vi "reset_trig.vi"(8 "error in (no error)":errorcluster, 11 "VISA resource name":refnum<visa-resource-name>) -> (0 "error out":errorcluster, 3 "VISA resource name out":refnum<visa-resource-name>)   [LabVIEW 2011]
doc: "This vi resets TRIG2 (DG645) to its defaultsetup and then configures a default setup for the chirped pulse setup.\nThis includes activating the burst mode (3 bursts, 100us burst period), setting polarities as well as setting all delays and durations to 0."
uses:
  global.vi
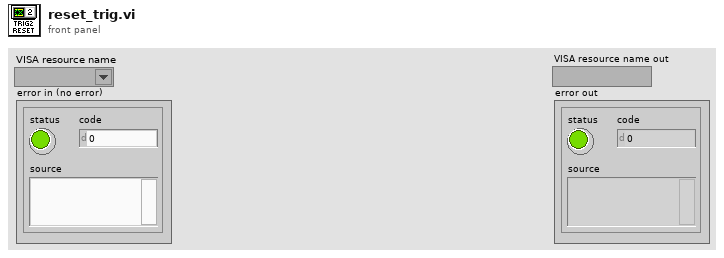
[diagram p1: front panel]
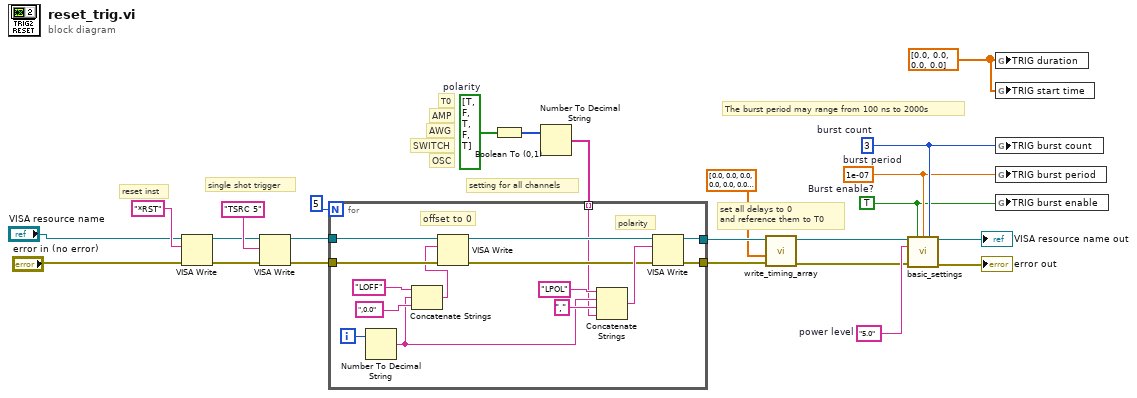
[diagram p0: block diagram]
diagram:
  w2 = bool[] [TRUE, FALSE, TRUE, FALSE, TRUE]  # polarity
  w5 = dbl[] [0.0, 0.0, 0.0, 0.0] ("duration")
  w12 = 3  # burst count
  w11 = 1e-07  # burst period
  w10 = TRUE  # Burst enable?
  w17 = "5.0"  # power level
  # "OSC"
  # "SWITCH"
  # "AWG"
  # "AMP"
  # "T0"
  # "The burst period may range from 100 ns to 2000s"
  # "set all delays to 0 \nand reference them to T0"
  # "reset inst"
  # "setting for all channels"
  # "single shot trigger"
  n1 = VISA Write(VISA resource name="VISA resource name", write buffer="*RST", error in (no error)="error in (no error)") -> (VISA resource name out=w19:refnum<visa-resource-name>, error out=w20:errorcluster)  [unwired: 1 out]
  n2 = VISA Write(VISA resource name=w19, write buffer="TSRC 5" ("Query 2"), error in (no error)=w20) -> (VISA resource name out=w22:refnum<visa-resource-name>, error out=w21:errorcluster)  [unwired: 1 out]
  n3 = Boolean To (0,1)(Boolean=w2) -> (0, 1=w3:i16[])
  n4 = Number To Decimal String(number=w3) -> (decimal integer string=w1:string[])  [unwired: 1 in]
  n5 = for {
    N: 5 -> [_]
    tunnel: w22 -> [w37]
    tunnel: [w28] -> w9
    tunnel: w21 -> [w36]
    tunnel: [w27] -> w8
    tunnel: w1 -> [w25] mode=indexing
    i -> [w35]
    # "polarity"
    # "offset to 0"
    n6 = Number To Decimal String(number=w35) -> (decimal integer string=w26:string)  [unwired: 1 in]
    n7 = Concatenate Strings("LOFF" ("Query 2"), w26, ",0.0" ("Query 2")) -> (w32:string)
    n8 = VISA Write(VISA resource name=w37, write buffer=w32, error in (no error)=w36) -> (VISA resource name out=w28:refnum<visa-resource-name>, error out=w27:errorcluster)  [unwired: 1 out]
    n9 = Concatenate Strings("LPOL" ("Query 2"), w26, "," ("string"), w25) -> (w30:string)
    n10 = VISA Write(VISA resource name=w28, write buffer=w30, error in (no error)=w27) -> ()  [unwired: 3 out]
  }
  n11 = call "write_timing_array.vi"("error in"=w8, "delay array"=dbl[] [0.0, 0.0, 0.0, 0.0, 0.0, 0.0, 0.0, 0.0] ("duration"), "VISA resource in"=w9) -> ("error out 2"=w6:errorcluster, "VISA resource out"=w7:refnum<visa-resource-name>)  [unwired: 3 in]
  n12 = call "basic_settings.vi"("VISA resource name"=w7, "Burst enable?"=w10, "burst period (s)"=w11, "burst count"=w12, "power level"=w17, "error in (no error)"=w6) -> ("VISA resource name out"=→"VISA resource name out":refnum<visa-resource-name>, "error out"=→"error out":errorcluster)  [unwired: 8 in]
  n13 = global write "global.vi" "TRIG duration"(w5) -> ()
  n14 = global write "global.vi" "TRIG start time"(w5) -> ()
  n15 = global write "global.vi" "TRIG burst count"(w12) -> ()
  n16 = global write "global.vi" "TRIG burst period"(w11) -> ()
  n17 = global write "global.vi" "TRIG burst enable"(w10) -> ()
